vi "AB_Engine_RESTful_Get_Supported_Classes.vi"() -> (2 "Web Request":string[](array[string]), 3 "Web Service":string[](array[string]))   [LabVIEW 2020]
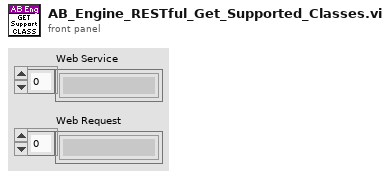
[diagram p1: front panel]
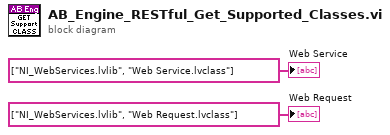
[diagram p0: block diagram]
diagram:
  "Web Request" <- string[] ["NI_WebServices.lvlib", "Web Request.lvclass"]
  "Web Service" <- string[] ["NI_WebServices.lvlib", "Web Service.lvclass"]
